vi "MidpointCalculate.vi"(9 "X2":dbl, 10 "X1":dbl) -> (2 "Midpoint":dbl)   [LabVIEW 2011]
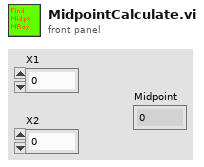
[diagram p1: front panel]
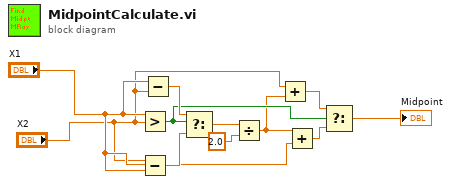
[diagram p0: block diagram]
diagram:
  n1 = Greater?(x="X1", y="X2") -> (0:w7:bool)
  n2 = Subtract(x="X2", y="X1") -> (x-y=w10:dbl)
  n3 = Subtract(x="X1", y="X2") -> (x-y=w11:dbl)
  n4 = Select(t=w11, s=w7, f=w10) -> (s? t:f=w9:dbl)
  n5 = Divide(x=w9, y=2.0) -> (x/y=w4:dbl)
  n6 = Add(x="X2", y=w4) -> (x+y=w6:dbl)
  n7 = Add(x=w4, y="X1") -> (x+y=w5:dbl)
  n8 = Select(t=w6, s=w7, f=w5) -> (s? t:f=→"Midpoint":dbl)
